vi "Report.vi"(8 "error in":errorcluster, 9 "Received":path, 10 "Approved":path, 11 "Report With DiffTool in":refnum<class "Report With DiffTool.lvclass">) -> (0 "error out":errorcluster, 2 "Worked?":bool, 3 "Report With DiffTool out":refnum<class "Report With DiffTool.lvclass">)   [LabVIEW 2020, in "Approval Tests.lvlib" / "Report With DiffTool.lvclass"]
uses:
  Report With DiffTool.lvclass
  C:/Users/SAS/Desktop/approval-testing/Approval Tests/Report With First Working/Report With First Working.lvclass
  Report With Beyord Compare/Report With Beyond Compare.lvclass
  C:/Users/SAS/Desktop/approval-testing/Approval Tests/Reporter/Reporter.lvclass
  Report Nothing/Report Nothing.lvclass
  Report With LVCompare/Report With LVCompare.lvclass
  Report With WinMerge/Report With WinMerge.lvclass
  Report With First Working/Report With First Working.lvclass/Report With First Working.ctl
  Report With First Working/Write Reporters.vi
  Report With First Working/Report With First Working.lvclass
  Report With DiffTool.lvclass/Report With DiffTool.ctl
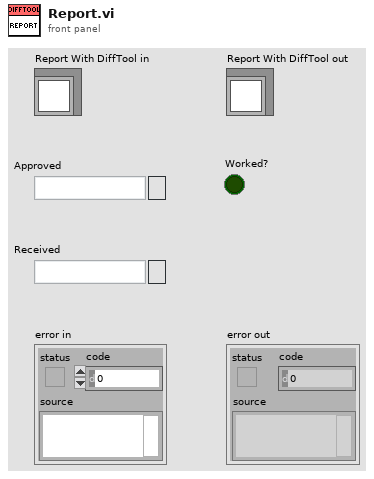
[diagram p1: front panel]
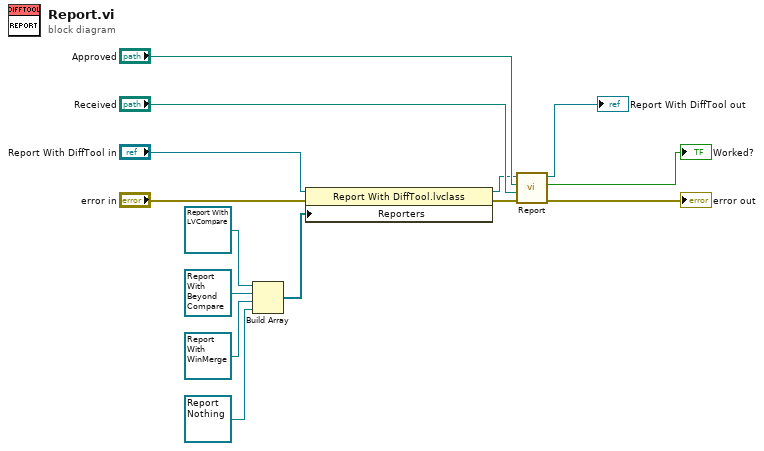
[diagram p0: block diagram]
diagram:
  n1 = Build Array(refnum<class "Report With LVCompare.lvclass"> refnum ("Approval Tests.lvlib:LVCompare.lvclass"), refnum<class "Report With Beyond Compare.lvclass"> refnum ("Approval Tests.lvlib:Beyond Compare.lvclass"), refnum<class "Report With WinMerge.lvclass"> refnum ("Approval Tests.lvlib:Report With WinMerge.lvclass"), refnum<class "Report Nothing.lvclass"> refnum ("Approval Tests.lvlib:Report Nothing.lvclass")) -> (w4:refnum<class "Reporter.lvclass">[])
  n2 = property class="Report With DiffTool.lvclass"(reference="Report With DiffTool in", error in="error in", "Reporters"=w4) -> (reference out=w6:refnum<class "Report With DiffTool.lvclass">, error out=w12:errorcluster)
  n3 = call-parent "Report.vi"("error in"=w12, "Received"="Received", "Approved"="Approved", "Report With First Working in"=w6) -> ("error out"=→"error out":errorcluster, "Worked?"=→"Worked?":bool, "Report With First Working out"=→"Report With DiffTool out":refnum<class "Report With DiffTool.lvclass">)  [unwired: 5 in]
